vi "classify error.vi"(8 "error to classify":errorcluster, 10 "attempt recovery?":bool, 11 "Shared Library Module runtime in":refnum<class "Shared Library Module runtime.lvclass">) -> (0 "classified error":errorcluster, 2 "error classification":T1, 3 "Shared Library Module runtime out":refnum<class "Shared Library Module runtime.lvclass">)   [LabVIEW 2013, in "Shared Library Module runtime.lvclass"]
doc: "Allows a module to classify an error generated at any point during execution. This <b>error classification</b> can then be used by calling code to determine if execution can continue. In addition, this function can be used to allow a component to clear an error, convert an error to a warning, or attempt to recover from an error. Recovery may be attempted only if <b>attempt recovery?</b> is true.Platypus Framework 1.0.1.60\nNI Systems Engineering - National Instruments"
uses:
  Shared Library Module runtime.lvclass
  <vilib>/NI/Tag Bus Module Framework/runtime/error classification.ctl
  Shared Library Module runtime.lvclass/Shared Library Module runtime.ctl
  <vilib>/NI/Tag Bus Module Framework/runtime/TBM module execution interface.lvclass
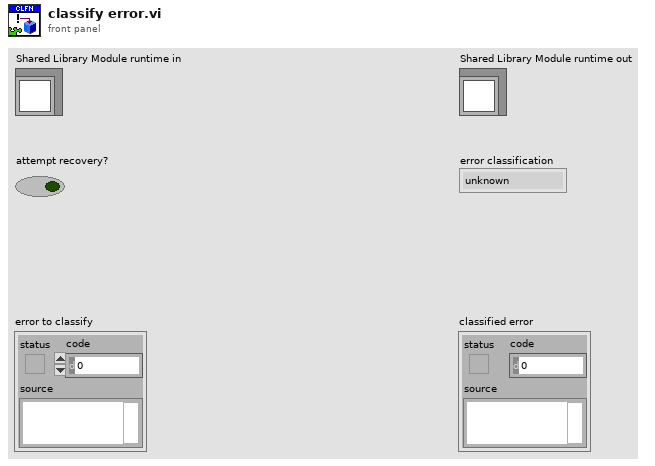
[diagram p1: front panel]
types:
  T1 = typedef "TBM module execution interface.lvclass/error classification.ctl" = enum16{"unknown", "none", "trivial", "recoverable", "critical"}
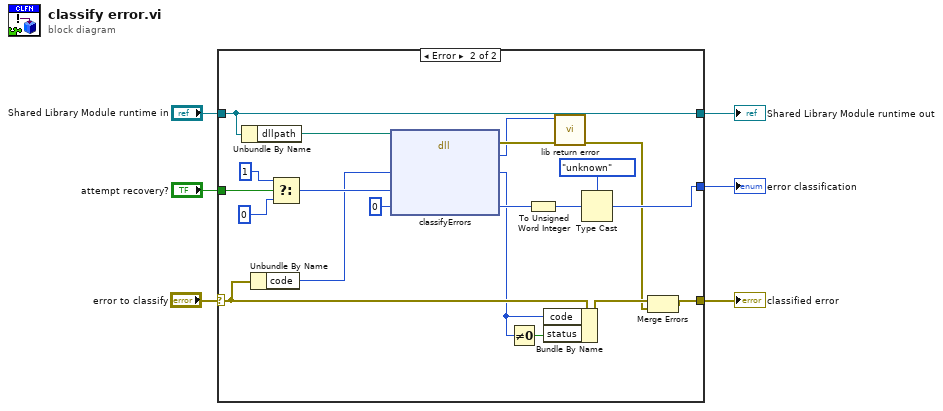
[diagram p0: block diagram]
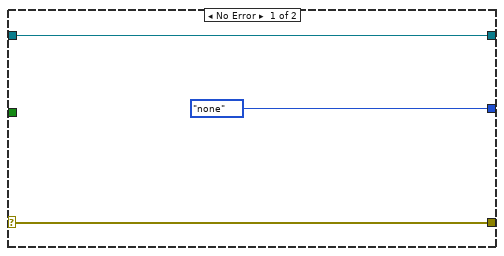
[diagram p2: hidden frame]
diagram:
  n1 = case shown="Error" "error to classify" {
    selector: "error to classify" -> [w7 w29]
    tunnel: "attempt recovery?" -> [_ w23]
    tunnel: [w8 w28] -> w2
    tunnel: "Shared Library Module runtime in" -> [w8 w28]
    tunnel: [w7 w25] -> w4
    tunnel: [error_classification."none" ("error classification") w16] -> w3
    frame No Error {
    }
    frame Error {
      n2 = Unbundle By Name(w28) -> ("dllpath"=w27:path)
      n3 = Unbundle By Name(w29) -> ("code"=w15:i32)
      n4 = Select(t=u8 1 ("bool"), s=w23, f=u8 0 ("bool")) -> (s? t:f=w21:u8)
      n5 = dll-call lib="?" fn="classifyErrors"(path in=w27, "err"=w15, "bool"=w21, "errtype"=u64 0) -> (error out=w12:errorcluster, "return type"=w10:i32, "err"=w13:i32, "errtype"=w19:u64)  [unwired: 3 in, 1 out]
      n6 = Not Equal To 0?(x=w13) -> (x != 0?=w14:bool)
      n7 = To Unsigned Word Integer(number=w19) -> (unsigned 16bit integer=w18:u16)
      n8 = Bundle By Name(cluster=w29, "code"=w13, "status"=w14) -> (w26:errorcluster)
      n9 = call "lib return error.vi"("error in"=w12, "return value"=w10) -> ("error out"=w11:errorcluster)  [unwired: 9 in]
      n10 = Type Cast(type=error_classification."unknown" ("error classification"), x=w18) -> (*(type *) &x=w16:T1)
      n11 = Merge Errors(w26, w11) -> (w25:errorcluster)
    }
  }
  "Shared Library Module runtime out" <- w2
  "error classification" <- w3
  "classified error" <- w4
